vi "Global_HW_Status.vi"() -> ()   [LabVIEW 2017, in "Intake.lvlib"]
uses:
  Intake.lvlib
  _SHARE ALL/RoboRio Share All/SRX Share All/TypeDefs SRX/Cluster_SRX_Common Runtime Data.ctl
  _SHARE ALL/RoboRio Share All/SRX Share All/TypeDefs SRX/Cluster_SRX_Error Calculations.ctl
  _SHARE ALL/RoboRio Share All/SRX Share All/TypeDefs SRX/Cluster_SRX_Voltage Out Data.ctl
  _SHARE ALL/RoboRio Share All/SRX Share All/TypeDefs SRX/Cluster_SRX_Sensor Out Data.ctl
panel:
  out "HW_Intake_Status":T1 {"Temp" format="%.1f"; "Voltage"."Bus" format="%.3f"; "Voltage"."Output" format="%.3f"; "Voltage"."Percent" format="%.3f"; "Current" format="%.2f"}
  # "C"
  # "Units"
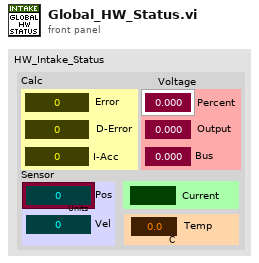
[diagram p1: front panel]
types:
  T1 = typedef "Cluster_SRX_Common Runtime Data.ctl" = cluster{"Calc":T2, "Voltage ":T3, "Sensor":T4, "Current":dbl, "Temp":dbl}
  T2 = typedef "Cluster_SRX_Error Calculations.ctl" = cluster{"Error":dbl, "D-Error":dbl, "I-Acc":dbl}
  T3 = typedef "Cluster_SRX_Voltage Out Data.ctl" = cluster{"Percent":dbl, "Output":dbl, "Bus":dbl}
  T4 = typedef "Cluster_SRX_Sensor Out Data.ctl" = cluster{"Pos":i32, "Vel":i32}
diagram:
